vi "Send Publish.vi"(6 "Publish Time (Use Current Time)":timestamp, 8 "error in (no error)":errorcluster, 9 "Data to Publish":variant, 10 "Topic Name":string, 11 "Publish Message":refnum<class "Publish Msg.lvclass">) -> (0 "error out":errorcluster, 3 "Message Enqueuer out":refnum<class "Message Enqueuer.lvclass">)   [LabVIEW 2015, in "IMediator.lvlib" / "Publish Msg.lvclass"]
doc: "This VI sends the message to an actor."
uses:
  Publish Msg.lvclass
  <vilib>/ActorFramework/Message Enqueuer/Message Enqueuer.lvclass
  AbstractMessages/PreAddressedMsg/PreAddressedMsg.lvclass/PreAddressedMsg.ctl
  Publish Msg.lvclass/Publish Msg.ctl
  <vilib>/ActorFramework/Message Enqueuer/Message Enqueuer.lvclass/Message Enqueuer.ctl
  <vilib>/ActorFramework/Message Priority Queue/Priority Enqueue.vi
  AbstractMessages/PreAddressedMsg/PreAddressedMsg.lvclass
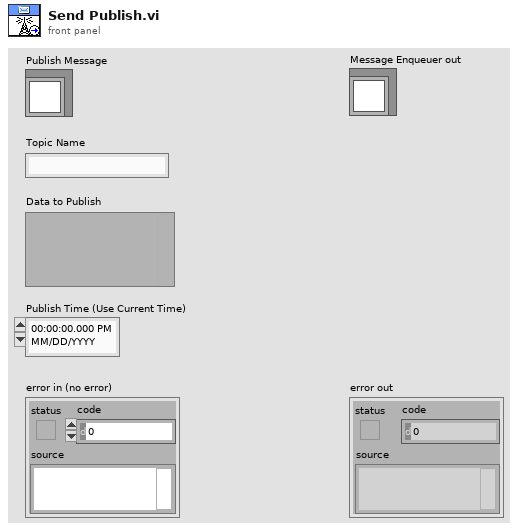
[diagram p1: front panel]
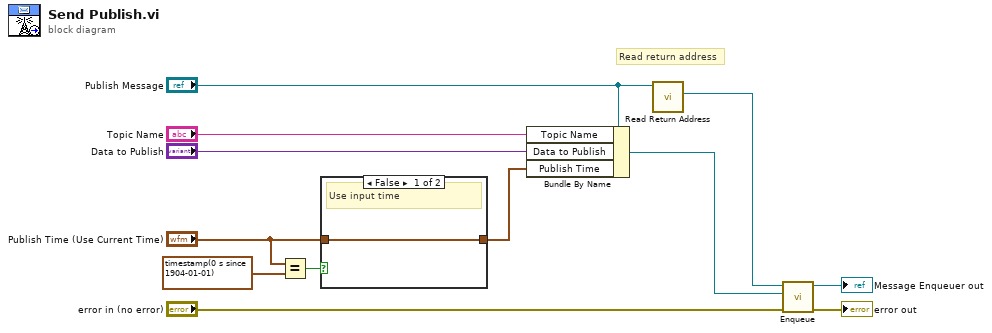
[diagram p0: block diagram]
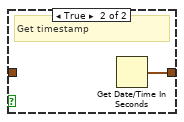
[diagram p2: hidden frame]
diagram:
  # "Read return address"
  n1 = Equal?(x="Publish Time (Use Current Time)", y=timestamp(0 s since 1904-01-01)) -> (x = y?=w2:bool)
  n2 = case shown="False" w2 {
    tunnel: "Publish Time (Use Current Time)" -> [w13 _]
    tunnel: [w13 w14] -> w4
    frame False {
      # "Use input time"
    }
    frame True {
      # "Get timestamp"
      n3 = Get Date/Time In Seconds() -> (seconds since 1Jan1904=w14:timestamp)
    }
  }
  n4 = Bundle By Name(cluster="Publish Message", "Topic Name"="Topic Name", "Data to Publish"="Data to Publish", "Publish Time"=w4) -> (w7:refnum<class "Publish Msg.lvclass">)
  n5 = call "Read Return Address.vi"("PreAddressedMsg in"="Publish Message") -> ("Return Address"=w5:refnum<class "Message Enqueuer.lvclass">)  [unwired: 9 in, 1 out]
  n6 = call <vilib>:"Enqueue.vi"("error in (no error)"="error in (no error)", "Message"=w7, "Message Enqueuer in"=w5) -> ("error out"=→"error out":errorcluster, "Message Enqueuer out"=→"Message Enqueuer out":refnum<class "Message Enqueuer.lvclass">)  [unwired: 7 in]
